vi "Path Graph Tester.vi"() -> ()   [LabVIEW 2016]
uses:
  <vilib>/Analysis/Matrix/Datatypes/RealMatrix.ctl
  <vilib>/Analysis/Matrix/NI_Matrix.lvlib
panel:
  out "Start Value by N":cluster{i32, "Radio Number":i32}[](graph)
  in  "Starting at N = ?":i32=2
  out "Finished?":bool
  out "Total time Progressed":u32
  out "Radio Number By N":cluster{i32, "Radio Number":i32}[](graph)
  out "Time By N":cluster{i32, "Run Time ms":u32}[](graph)
  in  "Up to N = ?":i32
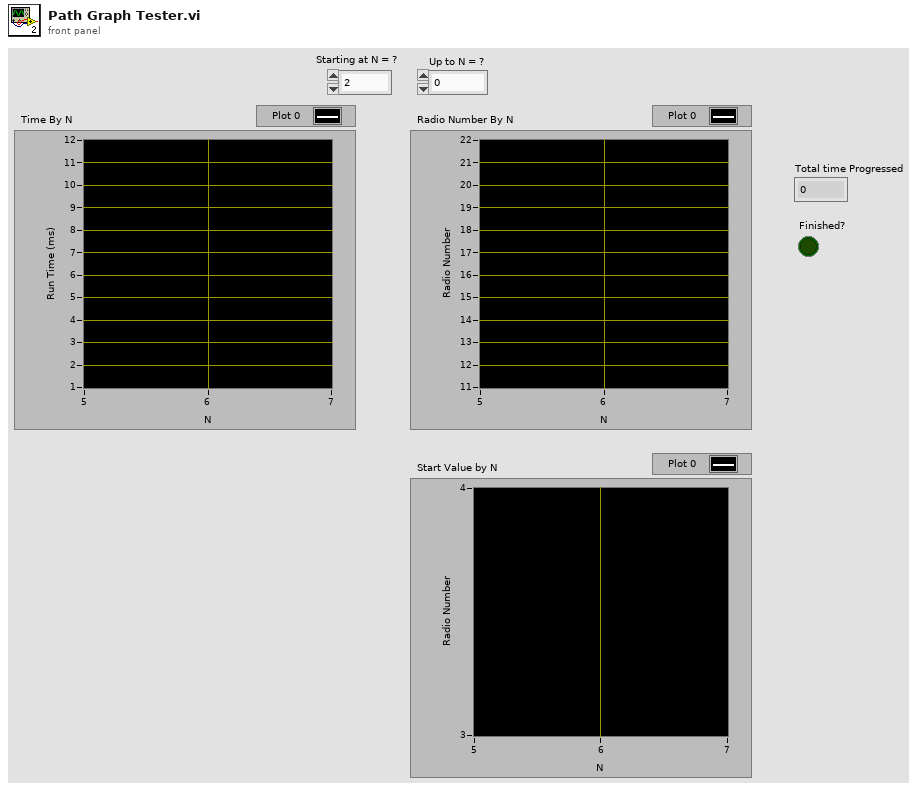
[diagram p1: front panel]
types:
  T1 = typedef "NI_Matrix.lvlib/RealMatrix.ctl" = dbl[][]
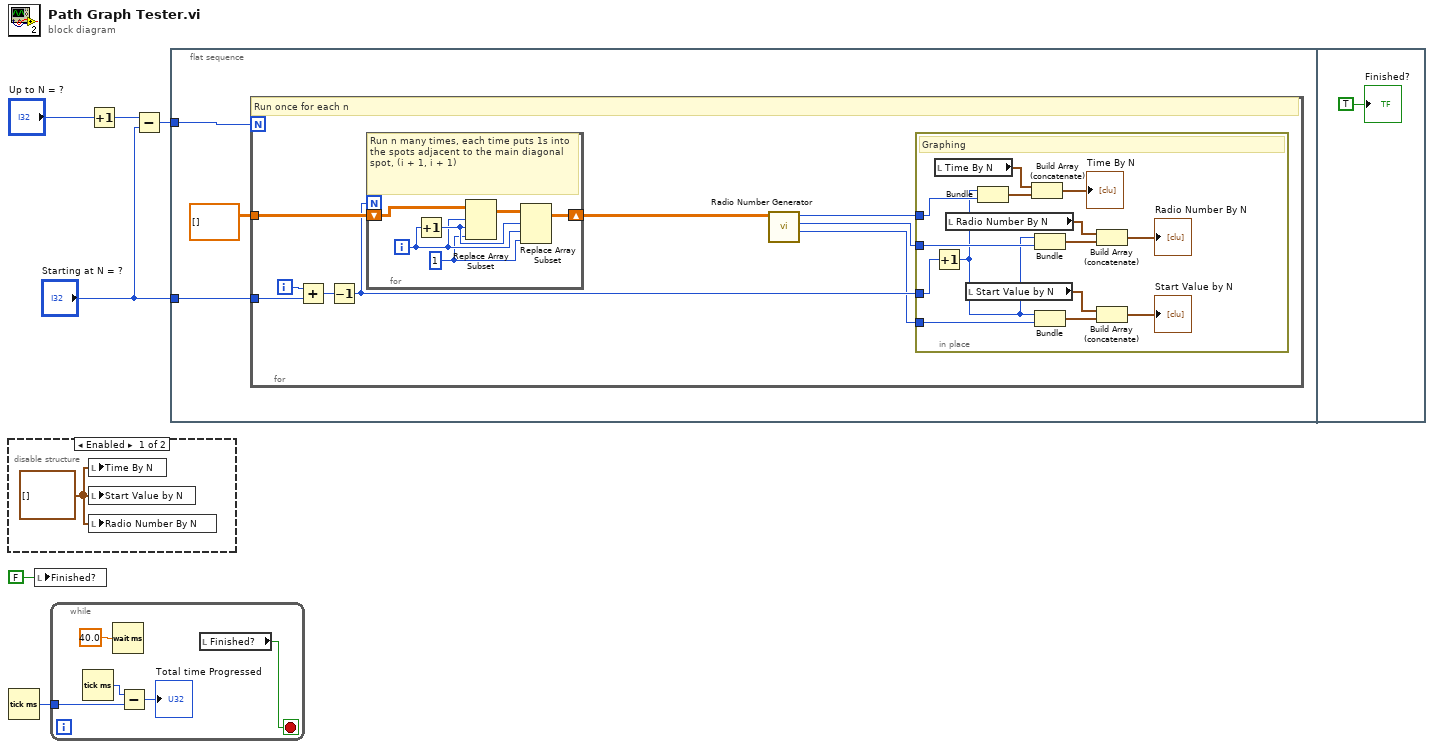
[diagram p0: block diagram]
diagram:
  n1 = disable-structure shown="Enabled" {
    frame Enabled {
      w7 = cluster{i32, "Radio Number":i32}[] [] ("appended array")
      n2 = local write "Time By N"(w7) -> ()
      n3 = local write "Start Value by N"(w7) -> ()
      n4 = local write "Radio Number By N"(w7) -> ()
    }
    frame Disabled {
    }
  }
  n5 = Tick Count (ms)() -> (millisecond timer value=w4:u32)
  n6 = local write "Finished?"(FALSE) -> ()
  n7 = while {
    tunnel: w4 -> [w9]
    stop <- w11 stop-if-true
    n8 = Tick Count (ms)() -> (millisecond timer value=w10:u32)
    n9 = Wait (ms)(milliseconds to wait=40.0) -> ()  [unwired: 1 out]
    n10 = Subtract(x=w10, y=w9) -> (x-y=→"Total time Progressed":u32)
    n11 = local read "Finished?"() -> (w11:bool)
  }
  n12 = Increment(x="Up to N = ?") -> (x+1=w1:i32)
  n13 = Subtract(x=w1, y="Starting at N = ?") -> (x-y=w5:i32)
  n14 = flat-sequence {
    tunnel: w5 -> [w14]
    tunnel: "Starting at N = ?" -> [w13]
    frame #0 {
      n15 = for {
        N: w14 -> [_]
        tunnel: T1 [] ("Adjacency Matrix") -> [w24]
        tunnel: w13 -> [w18]
        i -> [w23]
        # "Run once for each n"
        n16 = Add(x=w23, y=w18) -> (x+y=w20:i32)
        n17 = Decrement(x=w20) -> (x-1=w17:i32)
        n18 = for {
          N: w17 -> [_]
          shift-right: [w42] -> w22
          shift-left: w24 -> [w44]
          i -> [w40]
          w39 = 1
          # "Run n many times, each time puts 1s into the spots adjacent to the main diagonal spot, (i + 1, i + 1)"
          n19 = Increment(x=w40) -> (x+1=w41:i32)
          n20 = Replace Array Subset(array=w44, new element=w39, index (row)=w40, index (col)=w41) -> (w43:T1)
          n21 = Replace Array Subset(array=w43, new element=w39, index (row)=w41, index (col)=w40) -> (w42:T1)
        }
        n22 = call "Radio Number Generator.vi"("Adjacency Matrix"=w22) -> ("Start Value"=w16:i32, "Radio Number"=w21:i32, "Run Time ms"=w19:u32)  [unwired: 8 in]
        n23 = in-place {
          in-place-border: w21 -> [w38]
          in-place-border: w19 -> [w37]
          in-place-border: w17 -> [w30]
          in-place-border: w16 -> [w25]
          # "Graphing"
          n24 = Increment(x=w30) -> (x+1=w26:i32)
          n25 = local read "Time By N"() -> (w31:cluster{i32, "Run Time ms":u32}[])
          n26 = local read "Radio Number By N"() -> (w32:cluster{i32, "Radio Number":i32}[])
          n27 = local read "Start Value by N"() -> (w29:cluster{i32, "Radio Number":i32}[])
          n28 = Bundle(w26, "Run Time ms"=w37) -> (w36:cluster{i32, "Run Time ms":u32})  [unwired: 1 in]
          n29 = Build Array (concatenate)(w31, w36) -> (→"Time By N":cluster{i32, "Run Time ms":u32}[])
          n30 = Bundle(w26, "Radio Number"=w38) -> (w34:cluster{i32, "Radio Number":i32})  [unwired: 1 in]
          n31 = Bundle(w26, "Start Value"=w25) -> (w28:cluster{i32, "Start Value":i32})  [unwired: 1 in]
          n32 = Build Array (concatenate)(w32, w34) -> (→"Radio Number By N":cluster{i32, "Radio Number":i32}[])
          n33 = Build Array (concatenate)(w29, w28) -> (→"Start Value by N":cluster{i32, "Start Value":i32}[])
        }
      }
    }
    frame #1 {
      "Finished?" <- TRUE
    }
  }
